vi "SubVI_GenerateMatrixFSM300.vi"(0 "X center (Volt)":dbl, 1 "Total Length X (Volt)":dbl=1.0, 3 "''fast mooving'' axis":enum16{"Y", "X"}(ring), 4 "Y center (Volt)":dbl, 5 "Total Length Y (Volt)":dbl=1.0, 6 "Resolution X (Volt)":dbl=0.1, 7 "Resolution Y (Volt)":dbl=0.1, 11 "Scan mode":u16(ring)=4 items=["Default mode", "Snail mode", "Random mode", "Snake mode", "Line mode"]) -> (8 "XYPos Indices Randomized":dbl[][](array[numeric]), 9 "XYPos Indices":i32[][](array[numeric]), 10 "Y size":dbl=11.0, 12 "XYPositions":dbl[][](array[numeric])=[[-0.09999999999999998, -0.3], [-0.09999999999999998, -0.19999999999999996], [-0.3, 0.4], [0.20000000000000007, -0.09999999999999998], [-0.5, -0.5], [0.0, 0.20000000000000007], [0.30000000000000004, 0.30000000000000004], [-0.3, -0.5], [-0.5, 0.10000000000000009], [0.0, 0.4], [0.20000000000000007, 0.10000000000000009], [0.30000000000000004, 0.0], [-0.09999999999999998, -0.4], [-0.4, -0.19999999999999996], [-0.5, -0.19999999999999996], [0.4, 0.4], [-0.5, -0.4], [-0.5, -0.3], [-0.19999999999999996, 0.10000000000000009], [-0.19999999999999996, 0.4], [0.4, -0.5], [0.0, 0.10000000000000009], [-0.19999999999999996, 0.0], [0.10000000000000009, 0.30000000000000004], [-0.3, 0.10000000000000009], [0.10000000000000009, -0.3], [0.20000000000000007, -0.4], [-0.09999999999999998, 0.0], [-0.4, -0.5], [-0.5, 0.0], [-0.3, 0.20000000000000007], [-0.5, 0.20000000000000007], [-0.19999999999999996, 0.20000000000000007], [0.5, 0.4], [-0.4, 0.5], [0.5, 0.0], [0.5, 0.20000000000000007], [0.20000000000000007, -0.19999999999999996], [0.10000000000000009, -0.5], [0.4, 0.30000000000000004], [0.10000000000000009, 0.10000000000000009], [-0.4, 0.10000000000000009], [-0.5, 0.30000000000000004], [0.30000000000000004, -0.19999999999999996], [-0.09999999999999998, -0.5], [0.10000000000000009, -0.4], [0.20000000000000007, 0.5], [-0.3, -0.3], [0.4, 0.5], [0.30000000000000004, 0.5], [0.5, -0.3], [-0.09999999999999998, 0.30000000000000004], [0.10000000000000009, 0.20000000000000007], [0.5, 0.10000000000000009], [0.20000000000000007, 0.20000000000000007], [0.5, -0.5], [0.0, -0.5], [0.10000000000000009, 0.0], [0.10000000000000009, -0.19999999999999996], [-0.3, -0.19999999999999996], [-0.4, -0.09999999999999998], [0.20000000000000007, 0.30000000000000004], [0.20000000000000007, -0.5], [-0.3, 0.5], [0.4, 0.10000000000000009], [-0.3, -0.09999999999999998], [0.30000000000000004, -0.4], [0.30000000000000004, 0.10000000000000009], [0.30000000000000004, -0.3], [-0.4, 0.4], [0.5, -0.4], [-0.19999999999999996, -0.19999999999999996], [0.0, -0.19999999999999996], [0.4, 0.20000000000000007], [0.0, 0.0], [0.30000000000000004, 0.20000000000000007], [-0.09999999999999998, 0.5], [-0.3, -0.4], [0.4, -0.3], [0.0, 0.30000000000000004], [0.30000000000000004, 0.4], [0.0, -0.4], [-0.4, 0.30000000000000004], [0.20000000000000007, 0.4], [-0.5, 0.5], [-0.4, -0.4], [0.30000000000000004, -0.5], [0.10000000000000009, 0.4], [-0.09999999999999998, 0.10000000000000009], [0.10000000000000009, 0.5], [-0.4, -0.3], [0.5, -0.09999999999999998], [-0.5, -0.09999999999999998], [0.0, -0.09999999999999998], [-0.19999999999999996, -0.5], [0.4, 0.0], [0.0, -0.3], [-0.19999999999999996, 0.5], [0.5, -0.19999999999999996], [-0.09999999999999998, 0.20000000000000007], [-0.19999999999999996, -0.09999999999999998], [0.20000000000000007, 0.0], [-0.19999999999999996, 0.30000000000000004], [-0.19999999999999996, -0.3], [-0.5, 0.4], [0.10000000000000009, -0.09999999999999998], [-0.19999999999999996, -0.4], [-0.09999999999999998, 0.4], [0.30000000000000004, -0.09999999999999998], [-0.09999999999999998, -0.09999999999999998], [0.20000000000000007, -0.3], [-0.4, 0.20000000000000007], [0.4, -0.4], [-0.3, 0.30000000000000004], [0.5, 0.5], [0.4, -0.19999999999999996], [-0.3, 0.0], [0.0, 0.5], [0.5, 0.30000000000000004], [0.4, -0.09999999999999998], [-0.4, 0.0]], 13 "Random index":i32[](array[numeric])=[4, 16, 17, 14, 92, 29, 8, 31, 42, 104, 84, 28, 85, 90, 13, 60, 120, 41, 111, 82, 69, 34, 7, 77, 47, 59, 65, 116, 24, 30, 113, 2, 63, 94, 106, 103, 71, 100, 22, 18, 32, 102, 19, 97, 44, 12, 0, 1, 109, 27, 88, 99, 51, 107, 76, 56, 81, 96, 72, 93, 74, 21, 5, 79, 9, 117, 38, 45, 25, 58, 105, 57, 40, 52, 23, 87, 89, 62, 26, 110, 37, 3, 101, 10, 54, 61, 83, 46, 86, 66, 68, 43, 108, 11, 67, 75, 6, 80, 49, 20, 112, 78, 115, 119, 95, 64, 73, 39, 15, 48, 55, 70, 50, 98, 91, 35, 53, 36, 118, 33, 114], 14 "X0":dbl=-0.5, 15 "Xend":dbl=0.5, 16 "X size":dbl=11.0, 17 "Number of points":dbl=121.0, 18 "Y0":dbl=-0.5, 19 "Y end":dbl=0.5)   [LabVIEW 2019]
panel:
  in  "Blank Button":bool
  # "/!\\ Snake and snail mode not coded..."
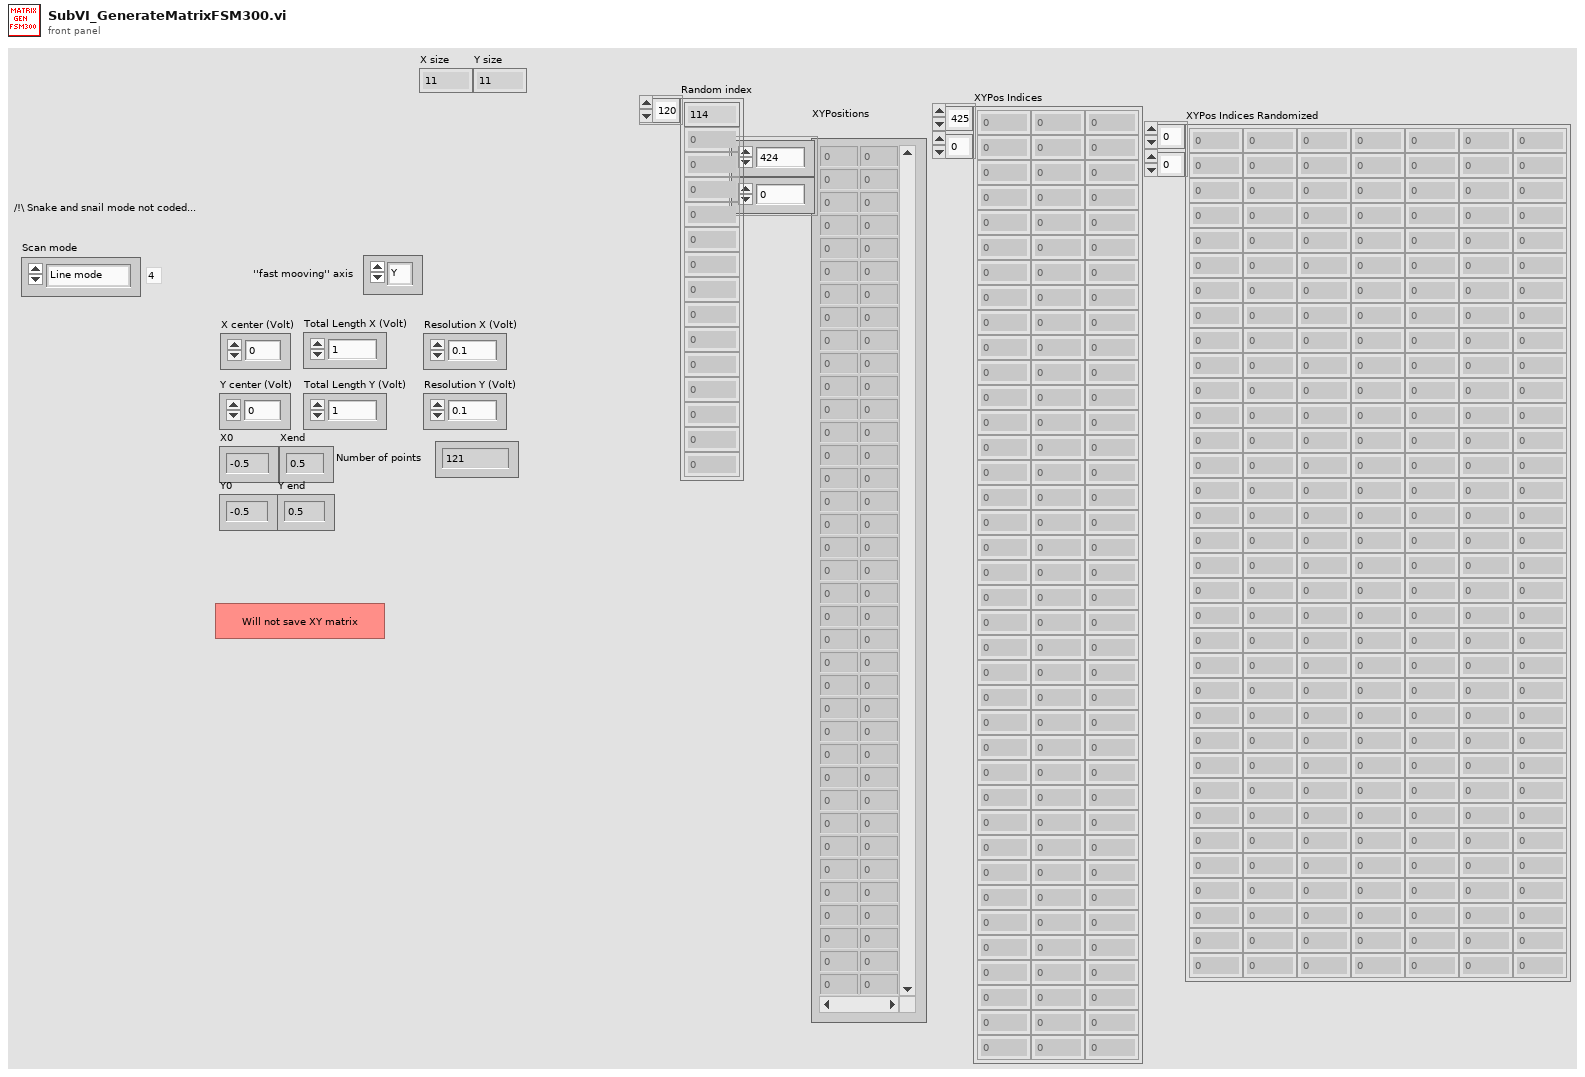
[diagram p1: front panel]
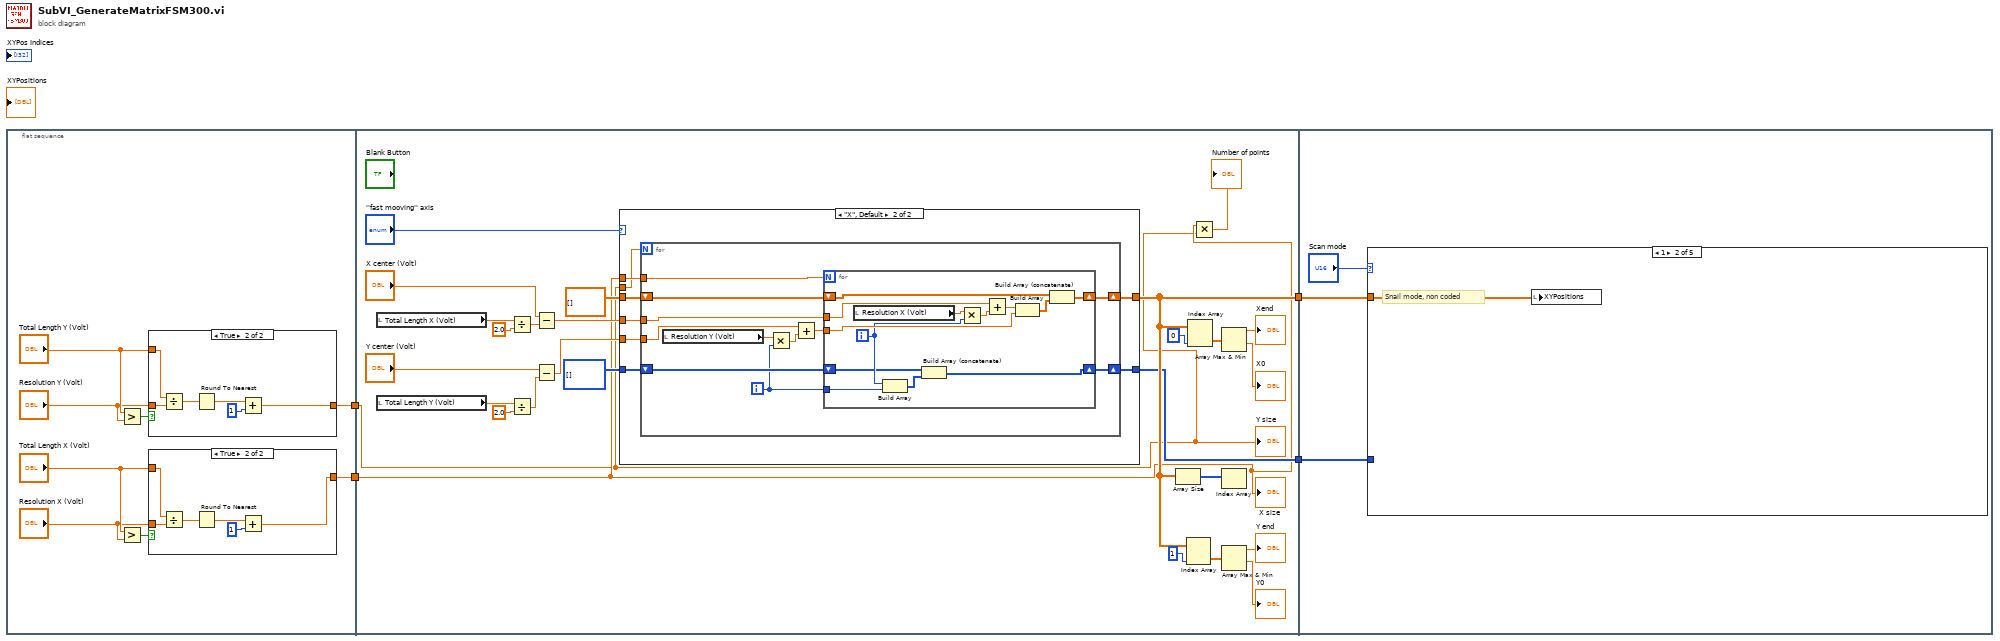
[diagram p0: block diagram]
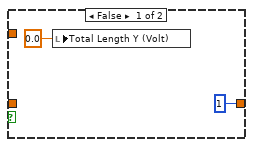
[diagram p2: hidden frame]
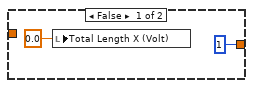
[diagram p3: hidden frame]
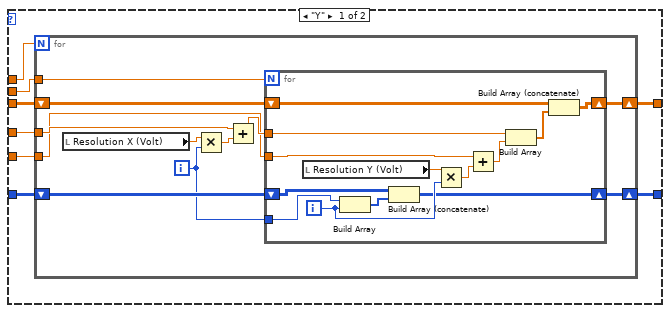
[diagram p4: hidden frame]
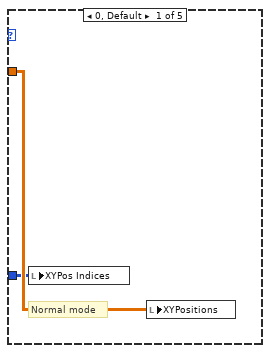
[diagram p5: hidden frame]
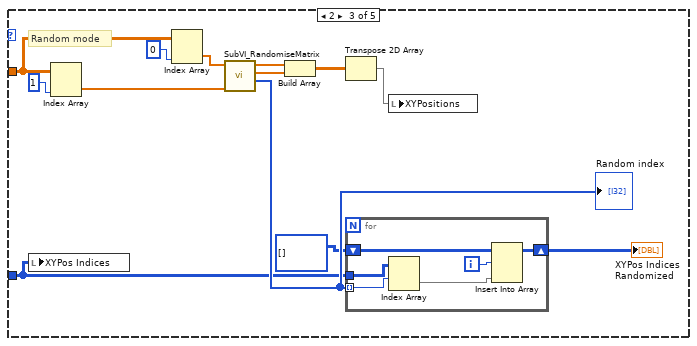
[diagram p6: hidden frame]
diagram:
  n1 = flat-sequence {
    tunnel: [w6] -> w4
    tunnel: [w5] -> w3
    tunnel: w4 -> [w31]
    tunnel: w3 -> [w30]
    tunnel: [w34] -> w2
    tunnel: [w32] -> w1
    tunnel: w2 -> [w122]
    tunnel: w1 -> [w120]
    frame #0 {
      n2 = Greater?(x="Total Length Y (Volt)", y="Resolution Y (Volt)") -> (0:w9:bool)
      n3 = Greater?(x="Total Length X (Volt)", y="Resolution X (Volt)") -> (0:w7:bool)
      n4 = case shown="True" w9 {
        tunnel: "Total Length Y (Volt)" -> [_ w18]
        tunnel: "Resolution Y (Volt)" -> [_ w17]
        tunnel: [1 w15] -> w5
        frame False {
          n5 = local write "Total Length Y (Volt)"(0.0 ("Total Length Y (Volt)")) -> ()
        }
        frame True {
          n6 = Divide(x=w18, y=w17) -> (x/y=w20:dbl)
          n7 = Round To Nearest(number=w20) -> (nearest integer value=w16:dbl)
          n8 = Add(x=w16, y=1) -> (x+y=w15:dbl)
        }
      }
      n9 = case shown="True" w7 {
        tunnel: "Total Length X (Volt)" -> [_ w28]
        tunnel: "Resolution X (Volt)" -> [_ w27]
        tunnel: [1 w23] -> w6
        frame False {
          n10 = local write "Total Length X (Volt)"(0.0 ("Total Length X (Volt)")) -> ()
        }
        frame True {
          n11 = Divide(x=w28, y=w27) -> (x/y=w26:dbl)
          n12 = Round To Nearest(number=w26) -> (nearest integer value=w24:dbl)
          n13 = Add(x=w24, y=1) -> (x+y=w23:dbl)
        }
      }
    }
    frame #1 {
      n14 = local read "Total Length X (Volt)"() -> (w40:dbl)
      n15 = local read "Total Length Y (Volt)"() -> (w39:dbl)
      n16 = Divide(x=w40, y=2.0) -> (x/y=w38:dbl)
      n17 = Divide(x=w39, y=2.0) -> (x/y=w37:dbl)
      n18 = Subtract(x="X center (Volt)", y=w38) -> (x-y=w36:dbl)
      n19 = Subtract(x="Y center (Volt)", y=w37) -> (x-y=w35:dbl)
      n20 = case shown="\"X\", Default" "''fast mooving'' axis" {
        tunnel: [w62 w95] -> w34
        tunnel: dbl[][] [] -> [w63 w94]
        tunnel: w36 -> [w61 w92]
        tunnel: w35 -> [w60 w93]
        tunnel: w31 -> [w59 w91]
        tunnel: w30 -> [w58 w90]
        tunnel: i32[][] [] -> [w57 w89]
        tunnel: [w56 w88] -> w32
        frame "Y" {
          n21 = for {
            N: w59 -> [_]
            shift-right: [w73] -> w62
            shift-left: w63 -> [w74]
            tunnel: w61 -> [w69]
            tunnel: w60 -> [w68]
            tunnel: w58 -> [w67]
            shift-right: [w64] -> w56
            shift-left: w57 -> [w66]
            i -> [w65]
            n22 = local read "Resolution X (Volt)"() -> (w72:dbl)
            n23 = Multiply(x=w72, y=w65) -> (x*y=w71:dbl)
            n24 = Add(x=w69, y=w71) -> (x+y=w70:dbl)
            n25 = for {
              N: w67 -> [_]
              shift-right: [w85] -> w73
              shift-left: w74 -> [w86]
              tunnel: w70 -> [w84]
              tunnel: w68 -> [w80]
              shift-right: [w75] -> w64
              shift-left: w66 -> [w77]
              tunnel: w65 -> [w79]
              i -> [w78]
              n26 = local read "Resolution Y (Volt)"() -> (w83:dbl)
              n27 = Build Array ("Construire un tableau")(w79, w78) -> (w76:i32[])
              n28 = Build Array (concatenate) ("Construire un tableau")(w77, w76) -> (w75:i32[][])
              n29 = Multiply(x=w83, y=w78) -> (x*y=w82:dbl)
              n30 = Add(x=w80, y=w82) -> (x+y=w81:dbl)
              n31 = Build Array ("Construire un tableau")(w84, w81) -> (w87:dbl[])
              n32 = Build Array (concatenate) ("Construire un tableau")(w86, w87) -> (w85:dbl[][])
            }
          }
        }
        frame "X", Default {
          n33 = for {
            N: w90 -> [_]
            shift-right: [w106] -> w95
            shift-left: w94 -> [w105]
            tunnel: w93 -> [w102]
            tunnel: w92 -> [w100]
            tunnel: w91 -> [w99]
            shift-right: [w97] -> w88
            shift-left: w89 -> [w98]
            i -> [w96]
            n34 = local read "Resolution Y (Volt)"() -> (w103:dbl)
            n35 = Multiply(x=w103, y=w96) -> (x*y=w104:dbl)
            n36 = Add(x=w102, y=w104) -> (x+y=w101:dbl)
            n37 = for {
              N: w99 -> [_]
              shift-right: [w112] -> w106
              shift-left: w105 -> [w119]
              tunnel: w101 -> [w118]
              tunnel: w100 -> [w115]
              shift-right: [w107] -> w97
              shift-left: w98 -> [w109]
              tunnel: w96 -> [w110]
              i -> [w111]
              n38 = local read "Resolution X (Volt)"() -> (w116:dbl)
              n39 = Build Array(w111, w110) -> (w108:i32[])
              n40 = Build Array (concatenate)(w109, w108) -> (w107:i32[][])
              n41 = Multiply(x=w116, y=w111) -> (x*y=w117:dbl)
              n42 = Add(x=w115, y=w117) -> (x+y=w114:dbl)
              n43 = Build Array ("Construire un tableau")(w114, w118) -> (w113:dbl[])
              n44 = Build Array (concatenate) ("Construire un tableau")(w119, w113) -> (w112:dbl[][])
            }
          }
        }
      }
      n45 = Array Size(array=w34) -> (size(s)=w51:i32[])
      n46 = Index Array(array=w34, index (col)=1) -> (element=w52:dbl[])  [unwired: 1 in]
      n47 = Index Array(array=w34, index (col)=0) -> (element=w53:dbl[])  [unwired: 1 in]
      n48 = Multiply(x=w31, y=w30) -> (x*y=→"Number of points":dbl)
      n49 = Array Max & Min(array=w53) -> (max value=→"Xend":dbl, min value=→"X0":dbl)  [unwired: 2 out]
      n50 = Index Array(array=w51) -> ()  [unwired: 1 in, 1 out]
      n51 = Array Max & Min(array=w52) -> (max value=→"Y end":dbl, min value=→"Y0":dbl)  [unwired: 2 out]
      "X size" <- w31
      "Y size" <- w30
    }
    frame #2 {
      n52 = case shown="1" "Scan mode" {
        tunnel: w122 -> [w124 w125 w137 _ _]
        tunnel: w120 -> [w123 _ w126 _ _]
        frame 0, Default {
          # "Normal mode"
          n53 = local write "XYPos Indices"(w123) -> ()
          n54 = local write "XYPositions"(w124) -> ()
        }
        frame 1 {
          # "Snail mode, non coded"
          n55 = local write "XYPositions"(w125) -> ()
        }
        frame 2 {
          # "Random mode"
          n56 = local write "XYPos Indices"(w126) -> ()
          n57 = Index Array(array=w137, index (col)=1 ("disabled index (col)")) -> (element=w134:dbl[])  [unwired: 1 in]
          n58 = Index Array(array=w137, index (col)=0 ("disabled index (col)")) -> (element=w135:dbl[])  [unwired: 1 in]
          n59 = call "SubVI_RandomiseMatrix.vi"("Y"=w134, "X"=w135) -> ("Random index"=w129:i32[], "Y shuffled"=w132:dbl[], "X shuffled"=w133:dbl[])  [unwired: 6 in, 1 out]
          "Random index" <- w129
          n60 = Build Array(w133, w132) -> (w131:dbl[][])
          n61 = Transpose 2D Array(2D array=w131) -> (transposed array=w130:dbl[][])
          n62 = for {
            tunnel: w129 -> [w143] mode=indexing
            tunnel: w126 -> [w144]
            shift-right: [w139] -> w127
            shift-left: i32[][] [] -> [w142]
            i -> [w141]
            n63 = Index Array(array=w144, index (row)=w143) -> (element=w140:i32[])  [unwired: 1 in]
            n64 = Insert Into Array(array=w142, index (row)=w141, new element=w140) -> (w139:i32[][])  [unwired: 1 in]
          }
          "XYPos Indices Randomized" <- w127
          n65 = local write "XYPositions"(w130) -> ()
        }
        frame 3 {
          # "Snake mode, non coded"
        }
        frame 4 {
          # "line mode"
        }
      }
    }
  }
